vi "Event Apply.vi"(8 "error in (no error)":errorcluster, 11 "[V] Sys Cfg Main in":refnum<class "[V] Sys Cfg Main.lvclass">) -> (0 "error out":errorcluster, 3 "[V] Sys Cfg Main out":refnum<class "[V] Sys Cfg Main.lvclass">)   [LabVIEW 2023, in "[V] Sys Cfg Main.lvlib" / "[V] Sys Cfg Main.lvclass"]
uses:
  [V] Sys Cfg Main.lvclass
  [V] Sys Cfg Main.lvclass/[V] Sys Cfg Main.ctl
  <vilib>/ActorFramework/Reply Msg/Reply Msg.lvclass/Reply Msg.ctl
  <vilib>/ActorFramework/Message Enqueuer/Message Enqueuer.lvclass/Message Enqueuer.ctl
  <vilib>/ActorFramework/Reply Msg/Send Message And Wait For Response.vi
  <vilib>/ActorFramework/Message Enqueuer/Enqueue.vi
  [V] Sys Cfg Base/[V] Sys Cfg Base Messages/Save Cfg File Msg/Save Cfg File Msg.lvclass
  C:/Program Files (x86)/National Instruments/LabVIEW 2023/vi.lib/ActorFramework/Reply Msg/Reply Msg.lvclass
  <vilib>/ActorFramework/Reply Msg/Reply Msg.lvclass
  C:/Program Files (x86)/National Instruments/LabVIEW 2023/vi.lib/ActorFramework/Message/Message.lvclass
  <vilib>/ActorFramework/Message Priority Queue/Priority Enqueue.vi
  Interface of [V] Sys Cfg Messages/[V] SC Update Msg/[V] SC Update Msg.lvclass
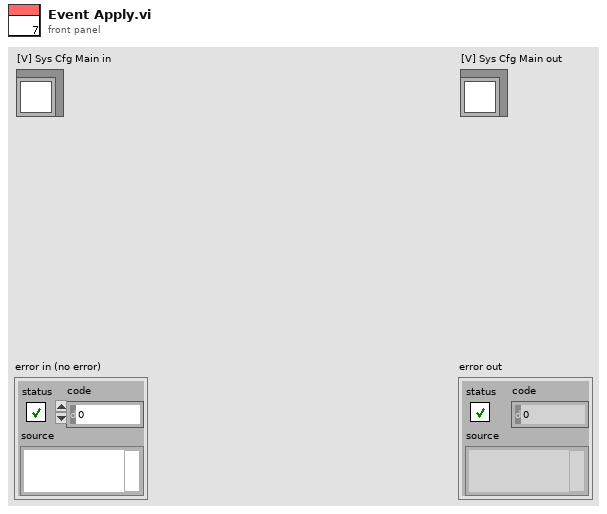
[diagram p1: front panel]
types:
  T1 = map{string, refnum<class "Message Enqueuer.lvclass">}
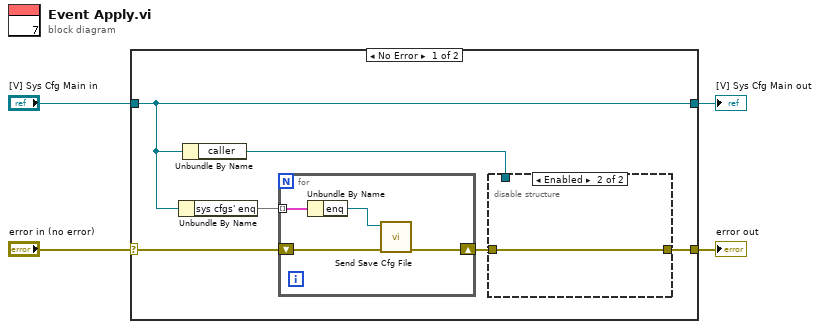
[diagram p0: block diagram]
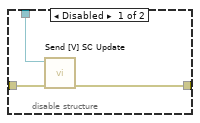
[diagram p2: hidden frame]
diagram:
  n1 = case shown="No Error" "error in (no error)" {
    selector: "error in (no error)" -> [w9 w20]
    tunnel: [w6 w20] -> w1
    tunnel: [w8 w19] -> w2
    tunnel: "[V] Sys Cfg Main in" -> [w8 w19]
    frame No Error {
      n2 = Unbundle By Name(w8) -> ("sys cfgs' enq"=w10:T1)
      n3 = Unbundle By Name(w8) -> ("caller"=w5:refnum<class "Message Enqueuer.lvclass">)
      n4 = for {
        tunnel: w10 -> [w18] mode=indexing
        shift-right: [w16] -> w7
        shift-left: w9 -> [w17]
        n5 = Unbundle By Name(w18) -> ("enq"=w15:refnum<class "Message Enqueuer.lvclass">)
        n6 = call "Send Save Cfg File.vi"("error in (no error)"=w17, "Message Enqueuer"=w15) -> ("error out"=w16:errorcluster)  [unwired: 6 in, 3 out]
      }
      n7 = disable-structure shown="Enabled" {
        disable-tunnel: w7 -> [w13 w14]
        disable-tunnel: [w12 w14] -> w6
        disable-tunnel: w5 -> [w11 _]
        frame Disabled {
          n8 = call "Send [V] SC Update.vi"("error in (no error)"=w13, "Message Enqueuer"=w11) -> ("error out"=w12:errorcluster)  [unwired: 8 in, 1 out]
        }
        frame Enabled {
        }
      }
    }
    frame Error {
    }
  }
  "error out" <- w1
  "[V] Sys Cfg Main out" <- w2
